vi "Test_Calculate CRT.vi"(8 "CRT_MAX":dbl, 9 "Time Data":dbl[](array[numeric]), 10 "Current Data":dbl[](array[numeric]), 11 "Piezo Data":dbl[](array[numeric])) -> (2 "Pass?":bool, 3 "CRT [ms]":dbl)   [LabVIEW 2025]
panel:
  out "T_0":dbl
  out "T_f":dbl
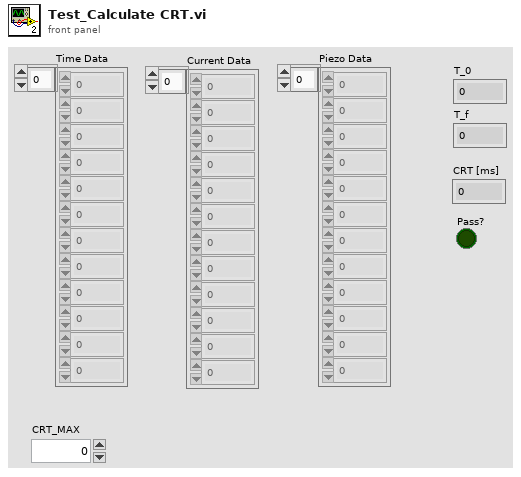
[diagram p1: front panel]
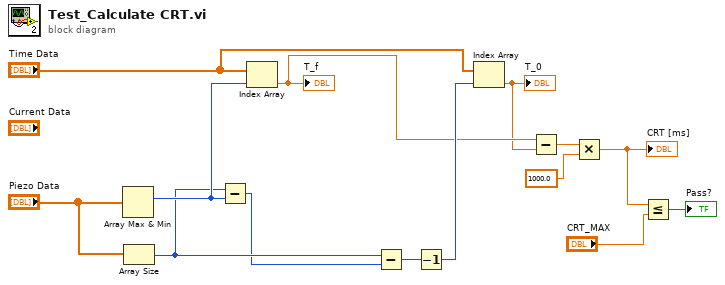
[diagram p0: block diagram]
diagram:
  n1 = Array Max & Min(array="Piezo Data") -> (max index (indices)=w13:i32)  [unwired: 3 out]
  n2 = Array Size(array="Piezo Data") -> (size(s)=w12:i32)
  n3 = Subtract(x=w12, y=w13) -> (x-y=w1:i32)
  n4 = Index Array(array="Time Data", index=w13) -> (element=w8:dbl)
  "T_f" <- w8
  n5 = Subtract(x=w12, y=w1) -> (x-y=w11:i32)
  n6 = Decrement(x=w11) -> (x-1=w9:i32)
  n7 = Index Array(array="Time Data", index=w9) -> (element=w7:dbl)
  "T_0" <- w7
  n8 = Subtract(x=w8, y=w7) -> (x-y=w6:dbl)
  n9 = Multiply(x=w6, y=1000.0) -> (x*y=w4:dbl)
  "CRT [ms]" <- w4
  n10 = Less Or Equal?(x=w4, y="CRT_MAX") -> (x <= y?=→"Pass?":bool)
